vi "getDeviceType.vi"(8 "error in (no error)":errorcluster, 11 "IDeviceInfo in":refnum<class "IDeviceInfo.lvclass">) -> (0 "error out":errorcluster, 2 "DeviceType out":refnum<class "IDeviceType.lvclass">, 3 "IDeviceInfo out":refnum<class "IDeviceInfo.lvclass">)   [LabVIEW 2022 SP3, in "openDAQ.lvlib" / "IBaseObject.lvlib" / "IPropertyObject.lvlib" / "IDeviceInfo.lvlib" / "IDeviceInfo.lvclass"]
uses:
  <instrlib>/openDAQ/Public/Classes/IDeviceInfo/IDeviceInfo.lvclass
  <instrlib>/openDAQ/Public/Classes/IDeviceInfo/IDeviceInfo.lvclass/IDeviceInfo.ctl
  <instrlib>/openDAQ/Public/Classes/IDeviceType/IDeviceType.lvclass
  <instrlib>/openDAQ/Binaries/Windows/x86/copendaq32.dll
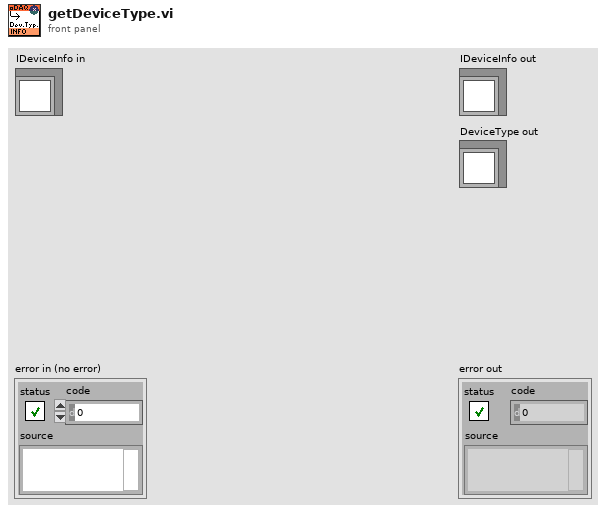
[diagram p1: front panel]
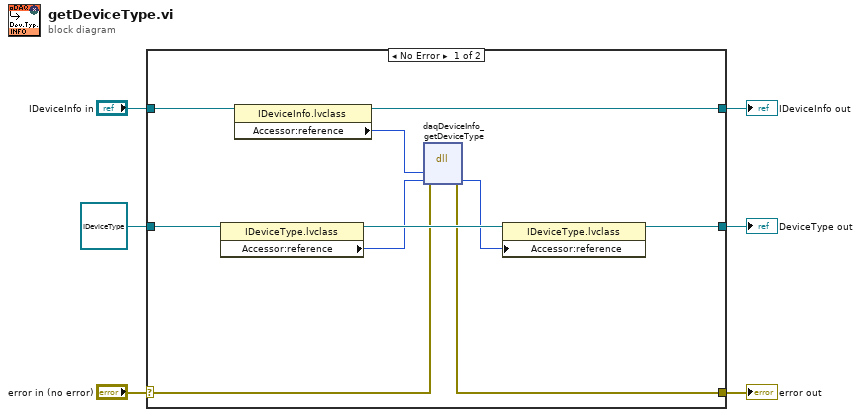
[diagram p0: block diagram]
diagram:
  n1 = case shown="No Error" "error in (no error)" {
    selector: "error in (no error)" -> [w9 w18]
    tunnel: [w7 w18] -> w5
    tunnel: [w13 w17] -> w3
    tunnel: "IDeviceInfo in" -> [w15 w17]
    tunnel: refnum<class "IDeviceType.lvclass"> refnum -> [w10 _]
    tunnel: [w8 _] -> w1
    frame No Error {
      n2 = property class="IDeviceType.lvclass"(reference=w10) -> (reference out=w16:refnum<class "IDeviceType.lvclass">, "Accessor:reference"=w12:i64)  [unwired: 1 in, 1 out]
      n3 = property class="IDeviceInfo.lvclass"(reference=w15) -> (reference out=w13:refnum<class "IDeviceInfo.lvclass">, "Accessor:reference"=w14:i64)  [unwired: 1 in, 1 out]
      n4 = dll-call lib="C:/Program Files (x86)/National Instruments/LabVIEW 2022/instr.lib/openDAQ/Binaries/Windows/x86/copendaq*.*" fn="daqDeviceInfo_getDeviceType"(error in=w9, "deviceInfo"=w14, "deviceType"=w12) -> (error out=w7:errorcluster, "deviceType"=w11:i64)  [unwired: 4 in, 1 out]
      n5 = property class="IDeviceType.lvclass"(reference=w16, "Accessor:reference"=w11) -> (reference out=w8:refnum<class "IDeviceType.lvclass">)  [unwired: 1 in, 1 out]
    }
    frame Error {
    }
  }
  "error out" <- w5
  "IDeviceInfo out" <- w3
  "DeviceType out" <- w1
